vi "FormatBias String.vi"(9 "current":dbl, 11 "bias":dbl) -> (2 "resulting string":string)   [LabVIEW 2014]
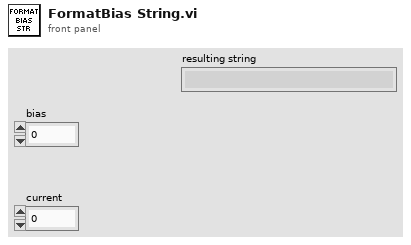
[diagram p1: front panel]
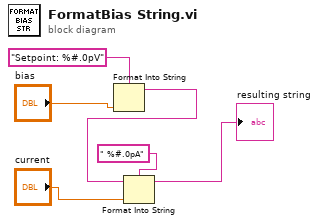
[diagram p0: block diagram]
diagram:
  n1 = Format Into String(format string="Setpoint: %#.0pV", "bias") -> (resulting string=w2:string)  [unwired: 2 in, 1 out]
  n2 = Format Into String(format string=" %#.0pA", initial string=w2, "current") -> (resulting string=→"resulting string":string)  [unwired: 1 in, 1 out]
